vi "K_S30c Terminal.vi"(4 "error in":errorcluster, 6 "request":u8[](array[numeric])) -> (0 "error out":errorcluster, 2 "response":u8[](array[numeric]))   [LabVIEW 2012]
uses:
  K_S30_VISA Global.vi
panel:
  in  "Case-Konstante\n(siehe Kontexthilfe)":bool
  out "msg and CRC":u8[](array[numeric])
  out "Echo":u8[](array[numeric])
  out "delited":u8[](array[numeric])
  # "Terminal for KELLER Transmitters Series3x \nVersion control:\nV1.0 15.11.2010  b.v. created\nV1.1 19.8.11 bv.MODBUS fct 1..16 & fct 20..23 added (for calibration only)\n\nConfigure ComPort: use K_S30 OpenComPort --> Global Variable\n\nsend a message with CRC16 checksum, receive the reponse\ncheck CRC16, and exceptions\n\nerrors:\n0: no error\n1,2,3,32: exceptions thrown by the device: see comm. protocol\n100: broadcast\n-2: wrong echo from the RS485 converter\n-4: timeout\n-5: CRC16 wrong\nothers thrown by VISA"
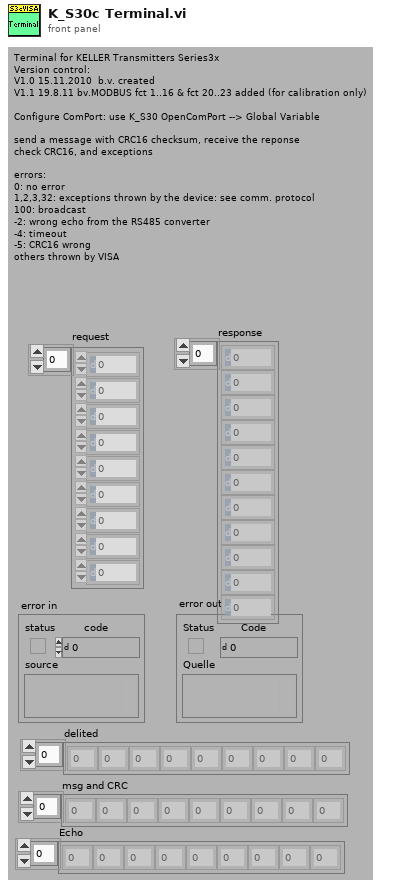
[diagram p1: front panel]
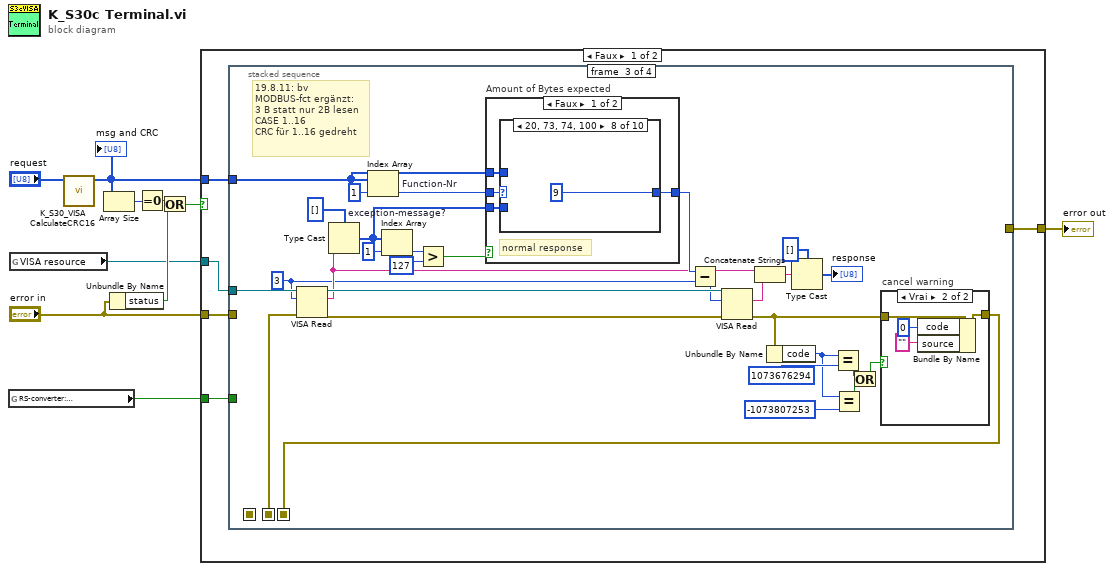
[diagram p0: block diagram]
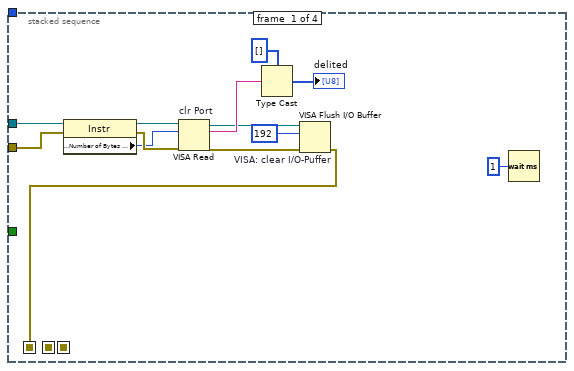
[diagram p2: hidden frame]
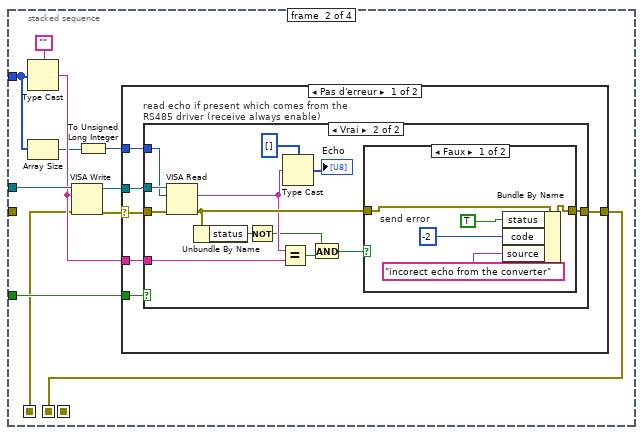
[diagram p3: hidden frame]
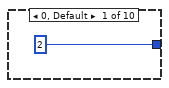
[diagram p8: hidden frame]
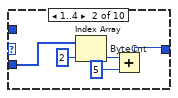
[diagram p9: hidden frame]
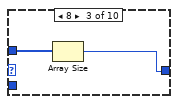
[diagram p10: hidden frame]
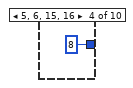
[diagram p11: hidden frame]
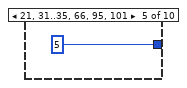
[diagram p12: hidden frame]
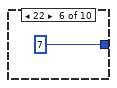
[diagram p13: hidden frame]
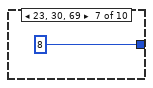
[diagram p14: hidden frame]
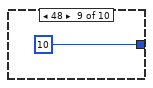
[diagram p15: hidden frame]
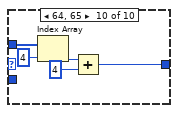
[diagram p16: hidden frame]
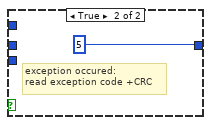
[diagram p17: hidden frame]
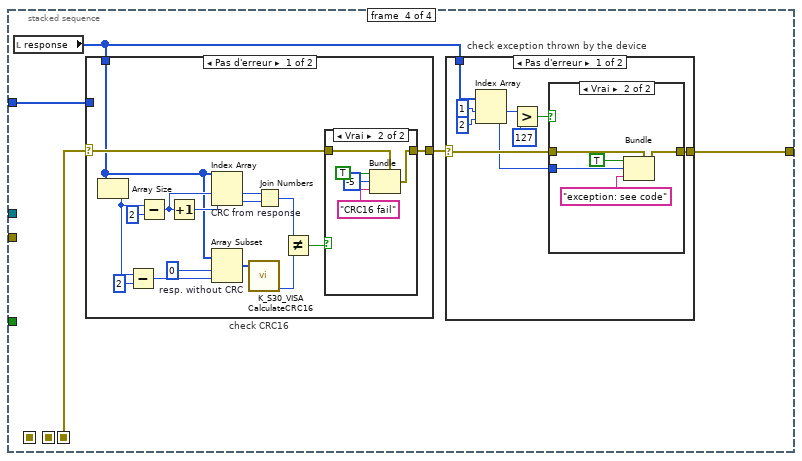
[diagram p18: hidden frame]
diagram:
  n1 = global read "K_S30_VISA Global.vi" "RS-converter:\necho"() -> (w2:bool)
  n2 = global read "K_S30_VISA Global.vi" "VISA resource"() -> (w1:refnum<visa-resource-name>)
  n3 = call "K_S30_VISA CalculateCRC16.vi"("msg without CRC"="request") -> ("msg and CRC"=w4:u8[])  [unwired: 3 in, 3 out]
  "msg and CRC" <- w4
  n4 = Array Size(array=w4) -> (size(s)=w5:i32)
  n5 = Unbundle By Name("error in") -> ("status"=w7:bool)
  n6 = Equal To 0?(x=w5) -> (x = 0?=w8:bool)
  n7 = Or(x=w8, y=w7) -> (x .or. y?=w6:bool)
  n8 = case shown="Faux" w6 {
    tunnel: w1 -> [w15 _]
    tunnel: "error in" -> [w14 w193]
    tunnel: w2 -> [w13 _]
    tunnel: w4 -> [w12 _]
    tunnel: [w11 w193] -> w3
    frame False {
      n9 = stacked-sequence {
        seq-local: [w18 _ _ _] -> [_ w30 _ _]
        seq-local: [_ w29 _ _] -> [_ _ w76 _]
        seq-local: [_ _ w77 _] -> [_ _ _ w126]
        tunnel: w15 -> [w16 w38 w94 _]
        tunnel: w14 -> [w24 _ _ _]
        tunnel: w13 -> [_ w37 _ _]
        tunnel: w12 -> [_ w34 w74 w125]
        tunnel: [_ _ _ w127] -> w11
        frame #0 {
          n10 = property class="Instr"(reference=w16, error in=w24) -> (reference out=w28:refnum<visa-resource-name>, error out=w27:errorcluster, "Serial Settings:Number of Bytes at Serial Port"=w26:u32)
          n11 = VISA Read "clr Port"(VISA resource name=w28, byte count=w26, error in (no error)=w27) -> (VISA resource name out=w20:refnum<visa-resource-name>, read buffer=w23:string, error out=w21:errorcluster)  [unwired: 1 out]
          n12 = Type Cast(type=u8[] [], x=w23) -> (*(type *) &x=→"delited":u8[])
          n13 = VISA Flush I/O Buffer "VISA: clear I/O-Puffer"(VISA resource name=w20, mask (16)=u16 192 ("Maskieren (16)"), error in (no error)=w21) -> (error out=w18:errorcluster)  [unwired: 1 out]
          n14 = Wait (ms)(milliseconds to wait=u32 1 ("ms Wartezeit")) -> ()  [unwired: 1 out]
        }
        frame #1 {
          n15 = Type Cast(type="", x=w34) -> (*(type *) &x=w35:string)
          n16 = Array Size(array=w34) -> (size(s)=w33:i32)
          n17 = VISA Write(VISA resource name=w38, write buffer=w35, error in (no error)=w30) -> (VISA resource name out=w39:refnum<visa-resource-name>, error out=w32:errorcluster)  [unwired: 1 out]
          n18 = To Unsigned Long Integer(number=w33) -> (unsigned 32bit integer=w31:u32)
          n19 = case shown="Pas d'erreur" w32 {
            selector: w32 -> [w40 w66]
            tunnel: w39 -> [w45 _]
            tunnel: w37 -> [w44 _]
            tunnel: [w43 w66] -> w29
            tunnel: w35 -> [w42 _]
            tunnel: w31 -> [w41 _]
            frame No Error {
              n20 = case "read echo if present which comes from the RS485 driver (receive always enable)" shown="Vrai" w44 {
                tunnel: w45 -> [_ w59]
                tunnel: w40 -> [w46 w58]
                tunnel: [w46 w53] -> w43
                tunnel: w42 -> [_ w57]
                tunnel: w41 -> [_ w47]
                frame False {
                }
                frame True {
                  n21 = VISA Read(VISA resource name=w59, byte count=w47, error in (no error)=w58) -> (read buffer=w52:string, error out=w56:errorcluster)  [unwired: 2 out]
                  n22 = Unbundle By Name(w56) -> ("status"=w55:bool)
                  n23 = Not(x=w55) -> (.not. x?=w49:bool)
                  n24 = Equal?(x=w52, y=w57) -> (x = y?=w48:bool)
                  n25 = Type Cast(type=u8[] [], x=w52) -> (*(type *) &x=→"Echo":u8[])
                  n26 = And(x=w49, y=w48) -> (x .and. y?=w54:bool)
                  n27 = case shown="Faux" w54 {
                    tunnel: w56 -> [w61 w65]
                    tunnel: [w60 w65] -> w53
                    frame False {
                      w62 = -2  # send error
                      n28 = Bundle By Name(cluster=w61, "status"=TRUE, "code"=w62, "source"="incorect echo from the converter") -> (w60:errorcluster)
                    }
                    frame True {
                    }
                  }
                }
              }
            }
            frame Error {
            }
          }
        }
        frame #2 {
          w75 = u32 3 ("Anzahl der Bytes (0)")
          # "19.8.11: bv\nMODBUS-fct ergänzt:\n3 B statt nur 2B lesen\nCASE 1..16\nCRC für 1..16 gedreht"
          n29 = VISA Read(VISA resource name=w94, byte count=w75, error in (no error)=w76) -> (VISA resource name out=w85:refnum<visa-resource-name>, read buffer=w82:string, error out=w86:errorcluster)  [unwired: 1 out]
          n30 = Type Cast(type=u8[] [], x=w82) -> (*(type *) &x=w73:u8[])
          n31 = Index Array "Function-Nr"(array=w74, index=1 ("Index")) -> (element=w88:u8)
          n32 = Index Array "exception-message?"(array=w73, index=1 ("Index")) -> (element=w92:u8)
          n33 = Greater?(x=w92, y=u8 127) -> (0:w90:bool)
          n34 = case "Amount of Bytes expected" shown="Faux" w90 {
            tunnel: w88 -> [w104 _]
            tunnel: [w103 u32 5] -> w87
            tunnel: w74 -> [w102 _]
            tunnel: w73 -> [w101 _]
            frame False {
              # "normal response"
              n35 = case shown="20, 73, 74, 100" w104 {
                tunnel: [u32 2 w106 w111 u32 8 u32 5 u32 7 u32 8 u32 9 u32 10 w119] -> w103
                tunnel: w102 -> [_ _ w112 _ _ _ _ _ _ w123]
                tunnel: w101 -> [_ w107 _ _ _ _ _ _ _ _]
                frame 0, Default {
                }
                frame 1..4 {
                  n36 = Index Array "ByteCnt"(array=w107, index=2 ("Index")) -> (element=w109:u8)
                  n37 = Add(x=w109, y=u8 5) -> (x+y=w106:u8)
                }
                frame 8 {
                  n38 = Array Size(array=w112) -> (size(s)=w111:i32)
                }
                frame 5, 6, 15, 16 {
                }
                frame 21, 31..35, 66, 95, 101 {
                }
                frame 22 {
                }
                frame 23, 30, 69 {
                }
                frame 20, 73, 74, 100 {
                }
                frame 48 {
                }
                frame 64, 65 {
                  n39 = Index Array(array=w123, index=4 ("Index")) -> (element=w121:u8)
                  n40 = Add(x=w121, y=u8 4) -> (x+y=w119:u8)
                }
              }
            }
            frame True {
              # "exception occured:\nread exception code +CRC"
            }
          }
          n41 = Subtract(x=w87, y=w75) -> (x-y=w84:u32)
          n42 = VISA Read(VISA resource name=w85, byte count=w84, error in (no error)=w86) -> (read buffer=w83:string, error out=w78:errorcluster)  [unwired: 2 out]
          n43 = Concatenate Strings(w82, w83) -> (w80:string)
          n44 = Unbundle By Name(w78) -> ("code"=w71:i32)
          n45 = Type Cast(type=u8[] [], x=w80) -> (*(type *) &x=→"response":u8[])
          n46 = Equal?(x=w71, y=1073676294 ("code")) -> (x = y?=w69:bool)
          n47 = Equal?(x=w71, y=-1073807253 ("code")) -> (x = y?=w68:bool)
          n48 = Or(x=w69, y=w68) -> (x .or. y?=w67:bool)
          n49 = case "cancel warning" shown="Vrai" w67 {
            tunnel: w78 -> [w96 w100]
            tunnel: [w96 w97] -> w77
            frame False {
            }
            frame True {
              n50 = Bundle By Name(cluster=w100, "code"=0, "source"="") -> (w97:errorcluster)
            }
          }
        }
        frame #3 {
          n51 = local read "response"() -> (w128:u8[])
          n52 = case "check CRC16" shown="Pas d'erreur" w126 {
            selector: w126 -> [w148 w172]
            tunnel: [w147 w171] -> w129
            tunnel: w128 -> [w146 _]
            tunnel: w125 -> [_ w168]
            frame No Error {
              n53 = Array Size(array=w146) -> (size(s)=w160:i32)
              n54 = Subtract(x=w160, y=2) -> (x-y=w158:i32)
              n55 = Subtract(x=w160, y=2) -> (x-y=w154:i32)
              n56 = Increment(x=w154) -> (x+1=w155:i32)
              n57 = Index Array "CRC from response"(array=w146, index #1=w154, index #2=w155) -> (element #1=w153:u8, element #2=w152:u8)
              n58 = Array Subset "resp. without CRC"(array=w146, index=0 ("Index"), length=w158) -> (w156:u8[])
              n59 = call "K_S30_VISA CalculateCRC16.vi"("msg without CRC"=w156) -> ("CRC16"=w150:u16)  [unwired: 3 in, 3 out]
              n60 = Join Numbers(hi=w153, lo=w152) -> ((hi.lo)=w151:u16)
              n61 = Not Equal?(x=w151, y=w150) -> (x != y?=w149:bool)
              n62 = case shown="Vrai" w149 {
                tunnel: w148 -> [w162 w164]
                tunnel: [w162 w163] -> w147
                frame False {
                }
                frame True {
                  n63 = Bundle(cluster=w164, "status"=TRUE, "code"=-5, "source"="CRC16 fail") -> (w163:errorcluster)
                }
              }
            }
            frame Error {
              w174 = -1073807339  # timeout
              n64 = Unbundle By Name(w172) -> ("code"=w175:i32)
              n65 = Index Array(array=w168, index=0 ("Index")) -> (element=w169:u8)
              n66 = Equal?(x=w175, y=w174) -> (x = y?=w173:bool)
              n67 = case shown="Vrai" w173 {
                tunnel: w172 -> [w176 w182]
                tunnel: [w176 w181] -> w171
                tunnel: w169 -> [_ w180]
                frame False {
                  # "other errors from VISA"
                  n68 = case shown="Vrai" "Case-Konstante\n(siehe Kontexthilfe)" {
                    tunnel: w176 -> [_ w178]
                    frame False {
                    }
                    frame True {
                      n69 = call <vilib>:"Simple Error Handler.vi"("error in (no error)"=w178) -> ()  [unwired: 4 in, 5 out]
                    }
                  }
                }
                frame True {
                  n70 = Equal To 0?(x=w180) -> (x = 0?=w179:bool)
                  n71 = case "Braoadcast?" shown="Vrai" w179 {
                    tunnel: w182 -> [w185 w189]
                    tunnel: [w184 w188] -> w181
                    frame False {
                      w183 = -4  # timeout
                      n72 = Bundle(cluster=w185, "status"=TRUE, "code"=w183, "source"="timeout") -> (w184:errorcluster)
                    }
                    frame True {
                      w190 = 100  # broadcast
                      n73 = Bundle(cluster=w189, "status"=TRUE, "code"=w190, "source"="broadcast") -> (w188:errorcluster)
                    }
                  }
                }
              }
            }
          }
          n74 = case "check exception thrown by the device" shown="Pas d'erreur" w129 {
            selector: w129 -> [w133 w145]
            tunnel: [w132 w145] -> w127
            tunnel: w128 -> [w135 _]
            frame No Error {
              n75 = Index Array(array=w135, index #1=1 ("Index"), index #2=2 ("Index")) -> (element #1=w137:u8, element #2=w130:u8)
              n76 = Greater?(x=w137, y=u8 127) -> (0:w134:bool)
              n77 = case shown="Vrai" w134 {
                tunnel: w133 -> [w139 w142]
                tunnel: [w139 w141] -> w132
                tunnel: w130 -> [_ w140]
                frame False {
                }
                frame True {
                  n78 = Bundle(cluster=w142, "status"=TRUE, "code"=w140, "source"="exception: see code") -> (w141:errorcluster)
                }
              }
            }
            frame Error {
            }
          }
        }
      }
    }
    frame True {
    }
  }
  "error out" <- w3
